vi "Script Data Control.vi"(4 "Message Paths":T5, 6 "Message":T1, 7 "App":refnum<vi>, 8 "error in (no error)":errorcluster, 11 "LV-Protoc in":refnum<class "LV-Protoc.lvclass">) -> (0 "error out":errorcluster, 3 "LV-Protoc out":refnum<class "LV-Protoc.lvclass">)   [LabVIEW 2020, in "LV-Protoc.lvlib" / "LV-Protoc.lvclass"]
uses:
  LV-Protoc.lvclass
  Message Paths.ctl
  LV-Proto/Message.ctl
  LV-Proto/Field.ctl
  LV-Proto/Type.ctl
  LV-Proto/Proto Type.ctl
  LV-Protoc.lvclass/LV-Protoc.ctl
  <vilib>/numeric/LVNumericRepresentation.ctl
  3e3d7e42-a8b8-4b7b-9c3f-59a4580cd892.vi
  Create Array Control.vi
  <vilib>/Comparison/Less/Less Functor/Less Functor.lvclass
  LV-Protoc.lvlib
  LV-Proto/LV-Proto.lvlib
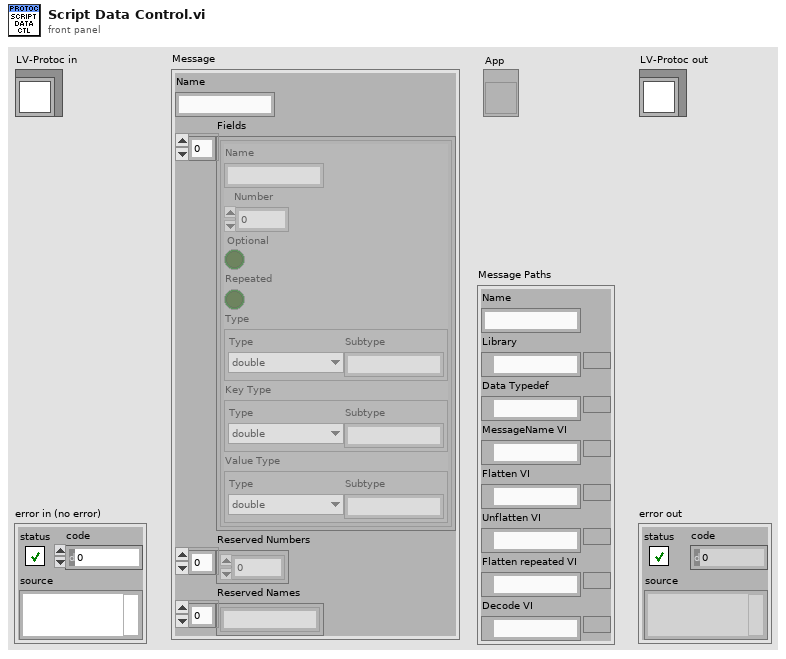
[diagram p1: front panel]
types:
  T1 = typedef "LV-Proto.lvlib/Message.ctl" = cluster{"Name":string, "Fields":T2[], "Reserved Numbers":u32[], "Reserved Names":string[]}
  T2 = typedef "LV-Proto.lvlib/Field.ctl" = cluster{"Name":string, "Number":u32, "Optional":bool, "Repeated":bool, "Type":T3, "Key Type":T3, "Value Type":T3}
  T3 = typedef "LV-Proto.lvlib/Type.ctl" = cluster{"Type":T4, "Subtype":string}
  T4 = typedef "LV-Proto.lvlib/Proto Type.ctl" = enum16{"UNKNOWN", "double", "float", "int32", "int64", "uint32", "uint64", "sint32", "sint64", "fixed32", "fixed64", "sfixed32", "sfixed64", "bool", "string", "bytes", "enum", "map", "message"}
  T5 = typedef "LV-Protoc.lvlib/Message Paths.ctl" = cluster{"Name":string, "Library":path, "Data Typedef":path, "MessageName VI":path, "Flatten VI":path, "Unflatten VI":path, "Flatten repeated VI":path, "Decode VI":path}
  T6 = typedef "LVNumericRepresentation.ctl" = enum32{"Extended Precision", "Double Precision", "Single Precision", "Long", "Word", "Byte", "Unsigned Long", "Unsigned Word", "Unsigned Byte", "Complex Extended", "Complex Double", "Complex Single", "Quad", "Unsigned Quad", "Fixed-Point"}
  T7 = typedef "LV-Protoc.lvlib/Enumeration Paths.ctl" = cluster{"Name":string, "Library":path, "Typedef":path, "Encode":path, "Encode packed":path, "Decode":path, "Decode packed":path, "Enum Value":path, "Enum from Value":path}
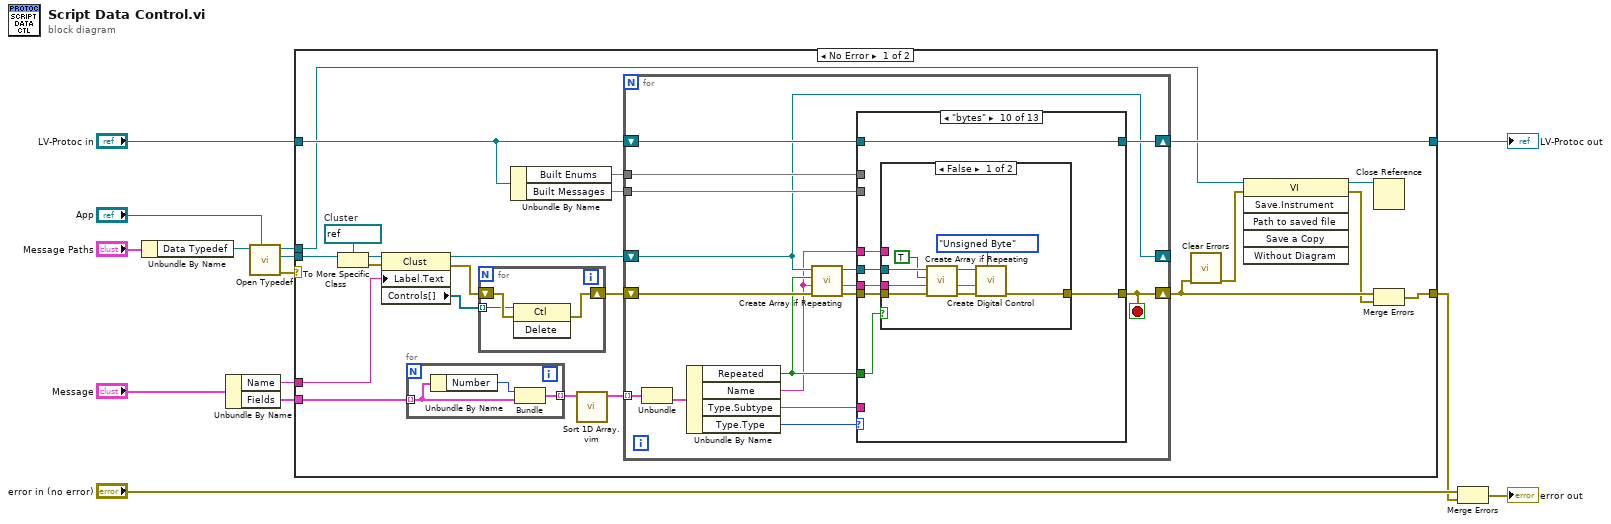
[diagram p0: block diagram]
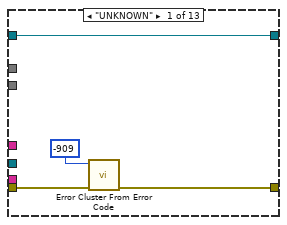
[diagram p2: hidden frame]
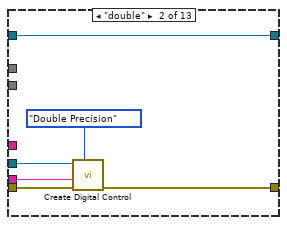
[diagram p3: hidden frame]
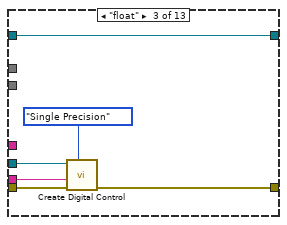
[diagram p4: hidden frame]
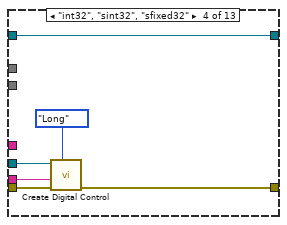
[diagram p5: hidden frame]
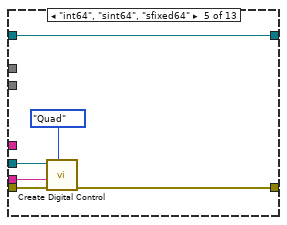
[diagram p6: hidden frame]
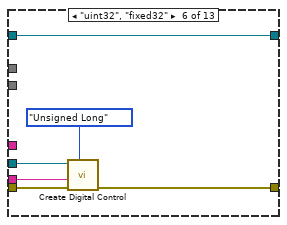
[diagram p7: hidden frame]
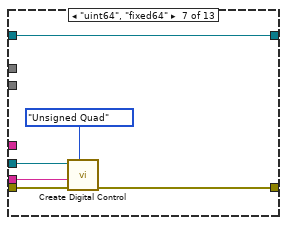
[diagram p8: hidden frame]
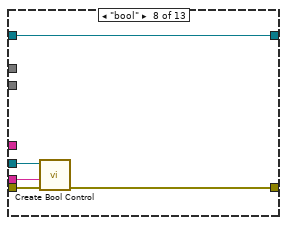
[diagram p9: hidden frame]
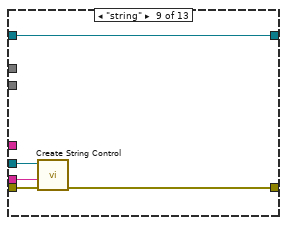
[diagram p10: hidden frame]
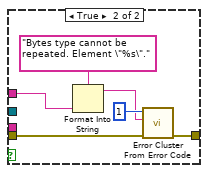
[diagram p11: hidden frame]
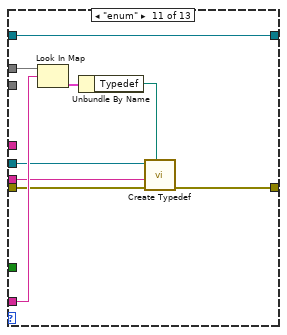
[diagram p12: hidden frame]
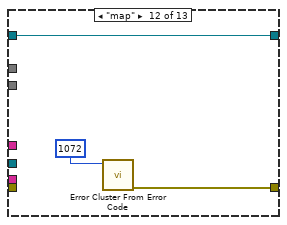
[diagram p13: hidden frame]
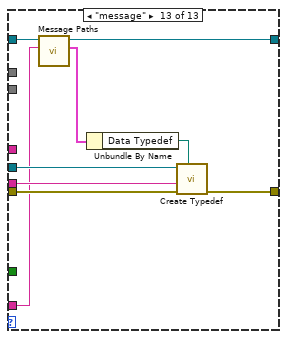
[diagram p14: hidden frame]
diagram:
  n1 = Unbundle By Name("Message Paths") -> ("Data Typedef"=w13:path)
  n2 = Unbundle By Name("Message") -> ("Name"=w7:string, "Fields"=w8:T2[])
  n3 = call "Open Typedef.vi"("App"="App", "Typedef Path"=w13) -> ("error out"=w12:errorcluster, "Control"=w11:refnum<vi>, "VI"=w10:refnum<vi>)  [unwired: 7 in]
  n4 = case shown="No Error" w12 {
    selector: w12 -> [_ w152]
    tunnel: w11 -> [w36 _]
    tunnel: w10 -> [w20 _]
    tunnel: w8 -> [w29 _]
    tunnel: w7 -> [w35 _]
    tunnel: "LV-Protoc in" -> [w23 w153]
    tunnel: [w24 w153] -> w5
    tunnel: [w16 w152] -> w2
    frame No Error {
      w33 = refnum<vi> refnum  # Cluster
      n5 = To More Specific Class(target class=w33, reference=w36) -> (specific class reference=w34:refnum<vi>, error out=w32:errorcluster)  [unwired: 1 in]
      n6 = property class="Clust"(reference=w34, error in=w32, "Label.Text"=w35) -> (reference out=w25:refnum<vi>, error out=w30:errorcluster, "Controls[]"=w31:refnum<vi>[])
      n7 = for {
        tunnel: w29 -> [w151] mode=indexing
        tunnel: [w149] -> w28 mode=indexing
        n8 = Unbundle By Name(w151) -> ("Number"=w150:u32)
        n9 = Bundle("Number"=w150, "Field"=w151) -> (w149:cluster{"Number":u32, "Field":T2})  [unwired: 1 in]
      }
      n10 = for {
        tunnel: w31 -> [w147] mode=indexing
        shift-right: [w146] -> w26
        shift-left: w30 -> [w148]
        n11 = invoke class="Ctl" method="Delete"(reference=w147, error in=w148) -> (error out=w146:errorcluster)  [unwired: 1 in, 2 out]
      }
      n12 = Unbundle By Name(w23) -> ("Built Enums"=w22:map{string, T7}, "Built Messages"=w21:map{string, T5})
      n13 = call "Sort 1D Array.vim"("unsorted array"=w28) -> ("sorted array"=w27:cluster{"Number":u32, "Field":T2}[])  [unwired: 10 in]
      n14 = for {
        tunnel: w27 -> [w52] mode=indexing
        shift-right: [w46] -> w19
        shift-left: w26 -> [w44]
        shift-right: [w38] -> _
        shift-left: w25 -> [w38]
        shift-right: [w49] -> w24
        shift-left: w23 -> [w50]
        tunnel: w22 -> [w48]
        tunnel: w21 -> [w47]
        stop <- w46 stop-if-true
        n15 = Unbundle(w52) -> ("Field"=w51:T2)  [unwired: 1 out]
        n16 = Unbundle By Name(w51) -> ("Repeated"=w39:bool, "Name"=w37:string, "Type.Subtype"=w45:string, "Type.Type"=w40:T4)
        n17 = call "Create Array if Repeating.vi"("error in (no error)"=w44, "Label"=w37, "Repeating"=w39, "Owner in"=w38) -> ("error out"=w41:errorcluster, "Nested Label"=w42:string, "Subcontrol Owner"=w43:refnum<vi>)  [unwired: 5 in]
        n18 = case shown="\"bytes\"" w40 {
          tunnel: w50 -> [w56 w62 w68 w74 w80 w86 w92 w97 w102 w109 w133 w136 w145]
          tunnel: [w56 w62 w68 w74 w80 w86 w92 w97 w102 w109 w133 w136 w144] -> w49
          tunnel: [w55 w61 w67 w73 w79 w85 w91 w96 w101 w104 w130 w134 w138] -> w46
          tunnel: w48 -> [_ _ _ _ _ _ _ _ _ _ w132 _ _]
          tunnel: w47 -> [_ _ _ _ _ _ _ _ _ _ _ _ _]
          tunnel: w45 -> [_ _ _ _ _ _ _ _ _ _ w128 _ w137]
          tunnel: w43 -> [_ w59 w65 w69 w75 w81 w87 w93 w98 w105 w127 _ w141]
          tunnel: w42 -> [_ w57 w64 w70 w76 w82 w88 w94 w99 w106 w126 _ w140]
          tunnel: w41 -> [w53 w58 w63 w71 w77 w83 w89 w95 w100 w108 w125 _ w142]
          tunnel: w39 -> [_ _ _ _ _ _ _ _ _ w107 _ _ _]
          tunnel: w37 -> [_ _ _ _ _ _ _ _ _ w103 _ _ _]
          frame "UNKNOWN" {
            n19 = call <vilib>:"Error Cluster From Error Code.vi"("error in (no error)"=w53, "error code (0)"=-909) -> ("error out"=w55:errorcluster)  [unwired: 7 in]
          }
          frame "double" {
            n20 = call "Create Digital Control.vi"("Numeric Representation"=LVNumericRepresentation."Double Precision" ("Representation"), "error in (no error)"=w58, "Label"=w57, "Owner in"=w59) -> ("error out"=w61:errorcluster)  [unwired: 6 in, 1 out]
          }
          frame "float" {
            n21 = call "Create Digital Control.vi"("Numeric Representation"=LVNumericRepresentation."Single Precision" ("Representation"), "error in (no error)"=w63, "Label"=w64, "Owner in"=w65) -> ("error out"=w67:errorcluster)  [unwired: 6 in, 1 out]
          }
          frame "int32", "sint32", "sfixed32" {
            n22 = call "Create Digital Control.vi"("Numeric Representation"=LVNumericRepresentation."Long" ("Representation"), "error in (no error)"=w71, "Label"=w70, "Owner in"=w69) -> ("error out"=w73:errorcluster)  [unwired: 6 in, 1 out]
          }
          frame "int64", "sint64", "sfixed64" {
            n23 = call "Create Digital Control.vi"("Numeric Representation"=LVNumericRepresentation."Quad" ("Representation"), "error in (no error)"=w77, "Label"=w76, "Owner in"=w75) -> ("error out"=w79:errorcluster)  [unwired: 6 in, 1 out]
          }
          frame "uint32", "fixed32" {
            n24 = call "Create Digital Control.vi"("Numeric Representation"=LVNumericRepresentation."Unsigned Long" ("Representation"), "error in (no error)"=w83, "Label"=w82, "Owner in"=w81) -> ("error out"=w85:errorcluster)  [unwired: 6 in, 1 out]
          }
          frame "uint64", "fixed64" {
            n25 = call "Create Digital Control.vi"("Numeric Representation"=LVNumericRepresentation."Unsigned Quad" ("Representation"), "error in (no error)"=w89, "Label"=w88, "Owner in"=w87) -> ("error out"=w91:errorcluster)  [unwired: 6 in, 1 out]
          }
          frame "bool" {
            n26 = call "Create Bool Control.vi"("error in (no error)"=w95, "Label"=w94, "Owner in"=w93) -> ("error out"=w96:errorcluster)  [unwired: 7 in, 1 out]
          }
          frame "string" {
            n27 = call "Create String Control.vi"("error in (no error)"=w100, "Label"=w99, "Owner in"=w98) -> ("error out"=w101:errorcluster)  [unwired: 7 in, 1 out]
          }
          frame "bytes" {
            n28 = case shown="False" w107 {
              tunnel: w108 -> [w115 w124]
              tunnel: w106 -> [w116 _]
              tunnel: w105 -> [w118 _]
              tunnel: [w110 w123] -> w104
              tunnel: w103 -> [_ w120]
              frame False {
                n29 = call "Create Array if Repeating.vi"("error in (no error)"=w115, "Label"=w116, "Repeating"=TRUE, "Owner in"=w118) -> ("error out"=w111:errorcluster, "Nested Label"=w112:string, "Subcontrol Owner"=w113:refnum<vi>)  [unwired: 5 in]
                n30 = call "Create Digital Control.vi"("Numeric Representation"=LVNumericRepresentation."Unsigned Byte" ("Representation"), "error in (no error)"=w111, "Label"=w112, "Owner in"=w113) -> ("error out"=w110:errorcluster)  [unwired: 6 in, 1 out]
              }
              frame True {
                n31 = Format Into String(format string="Bytes type cannot be repeated. Element \"%s\".", w120) -> (resulting string=w121:string)  [unwired: 2 in, 1 out]
                n32 = call <vilib>:"Error Cluster From Error Code.vi"("error in (no error)"=w124, "error message (\"\")"=w121, "error code (0)"=1) -> ("error out"=w123:errorcluster)  [unwired: 6 in]
              }
            }
          }
          frame "enum" {
            n33 = Look In Map(map=w132, key=w128) -> (value=w131:T7)  [unwired: 1 in, 1 out]
            n34 = Unbundle By Name(w131) -> ("Typedef"=w129:path)
            n35 = call "Create Typedef.vi"("Typedef Path"=w129, "error in (no error)"=w125, "Label"=w126, "Owner in"=w127) -> ("error out"=w130:errorcluster)  [unwired: 6 in, 1 out]
          }
          frame "map" {
            n36 = call <vilib>:"Error Cluster From Error Code.vi"("error code (0)"=1072) -> ("error out"=w134:errorcluster)  [unwired: 8 in]
          }
          frame "message" {
            n37 = call "Message Paths.vi"("Message Type Name"=w137, "LV-Protoc in"=w145) -> ("Message Paths"=w143:T5, "LV-Protoc out"=w144:refnum<class "LV-Protoc.lvclass">)  [unwired: 7 in, 1 out]
            n38 = Unbundle By Name(w143) -> ("Data Typedef"=w139:path)
            n39 = call "Create Typedef.vi"("Typedef Path"=w139, "error in (no error)"=w142, "Label"=w140, "Owner in"=w141) -> ("error out"=w138:errorcluster)  [unwired: 6 in, 1 out]
          }
        }
      }
      n40 = call <vilib>:"Clear Errors.vi"("error in (no error)"=w19) -> ("error out"=w18:errorcluster)  [unwired: 5 in, 1 out]
      n41 = invoke class="VI" method="Save.Instrument"(reference=w20, error in=w18) -> (reference out=w17:refnum<vi>, error out=w15:errorcluster)  [unwired: 4 in, 4 out]
      n42 = Close Reference(reference=w17) -> ()  [unwired: 1 in, 1 out]
      n43 = Merge Errors(w19, w15) -> (w16:errorcluster)
    }
    frame Error {
    }
  }
  "LV-Protoc out" <- w5
  n44 = Merge Errors("error in (no error)", w2) -> (→"error out":errorcluster)
